vi "Calculate Repeatability.vi"(8 "error in (no error)":errorcluster, 9 "SensorID":i32, 10 "FS Sensors":T1[](array[typedef]), 11 "Calibration Points":T3[](array[typedef])) -> (0 "error out":errorcluster, 2 "Max Repeatability":dbl, 3 "Repeatability Results":T2[](array[typedef]))   [LabVIEW 2026, in "Analysis.lvlib"]
uses:
  Analysis.lvlib
  controls/Messaging Payloads/Calibration Point Table Insert.ctl
  Repeatability Result.ctl
  Full Scale Sensor Cluster.ctl
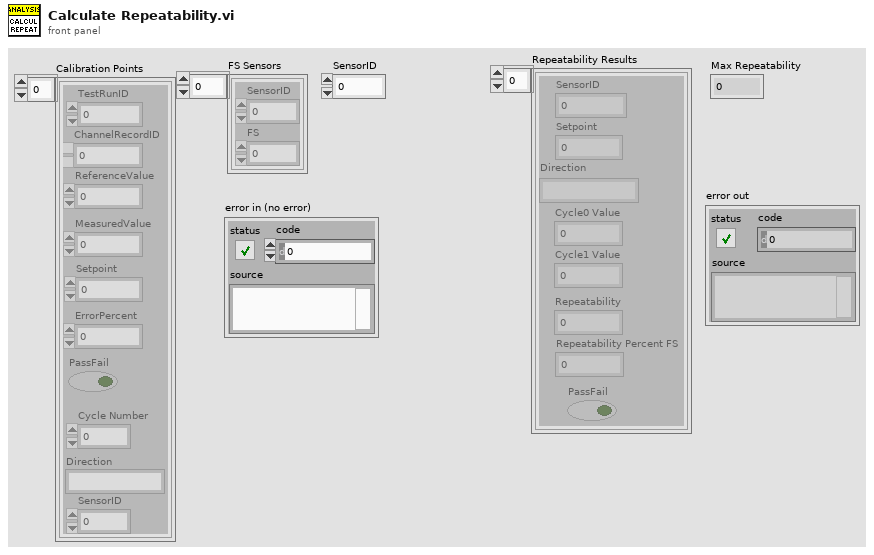
[diagram p1: front panel]
types:
  T1 = typedef "Analysis.lvlib/Full Scale Sensor Cluster.ctl" = cluster{"SensorID":i32, "FS":dbl}
  T2 = typedef "Analysis.lvlib/Repeatability Result.ctl" = cluster{"Setpoint":dbl, "Cycle0 Value":dbl, "SensorID":i32, "Cycle1 Value":dbl, "Repeatability":dbl, "Direction":string, "Repeatability Percent FS":dbl, "PassFail":bool}
  T3 = typedef "Calibration Point Table Insert.ctl" = cluster{"TestRunID":i32, "ChannelRecordID":i32, "Setpoint":dbl, "MeasuredValue":dbl, "ErrorPercent":dbl, "PassFail":bool, "ReferenceValue":dbl, "Cycle Number":i32, "Direction":string, "SensorID":i32}
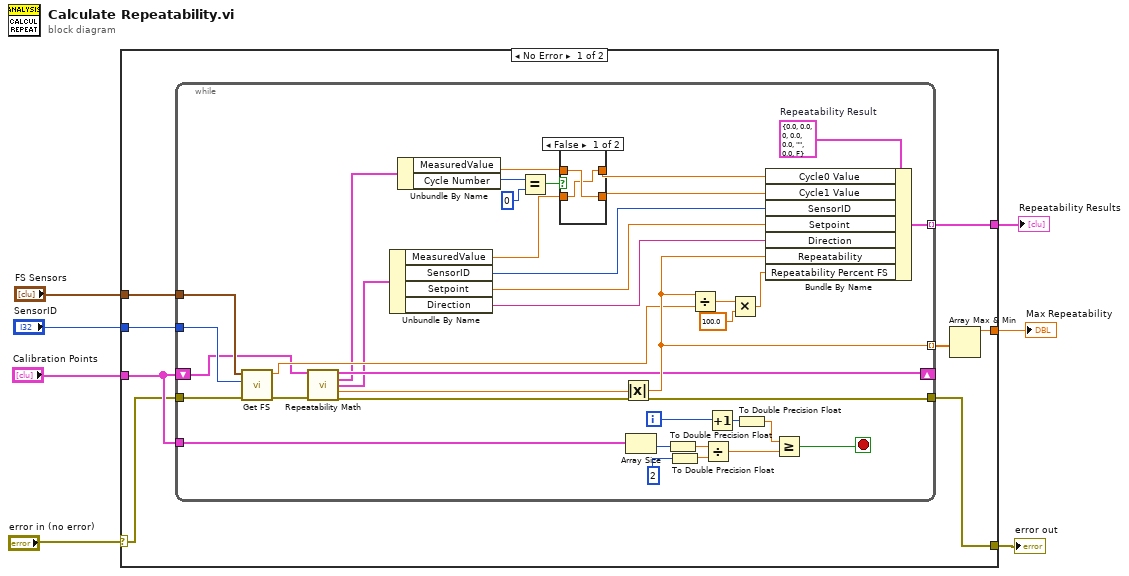
[diagram p0: block diagram]
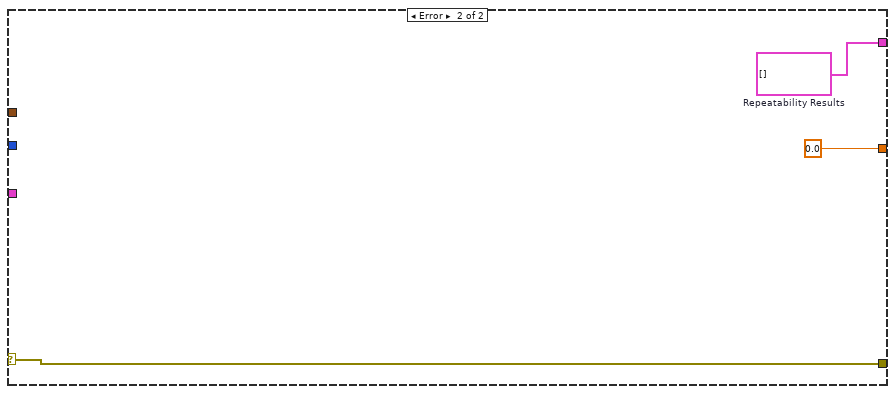
[diagram p3: hidden frame]
diagram:
  n1 = case shown="No Error" "error in (no error)" {
    selector: "error in (no error)" -> [w9 w59]
    tunnel: "Calibration Points" -> [w15 _]
    tunnel: [w8 w59] -> w5
    tunnel: [w14 w58] -> w4
    tunnel: [w12 0.0] -> w3
    tunnel: "FS Sensors" -> [w11 _]
    tunnel: "SensorID" -> [w10 _]
    frame No Error {
      n2 = while {
        shift-right: [w25] -> _
        shift-left: w15 -> [w21]
        tunnel: w15 -> [w43]
        tunnel: [w33] -> w14 mode=indexing
        tunnel: [w27] -> w13 mode=indexing
        tunnel: w11 -> [w32]
        tunnel: w10 -> [w31]
        tunnel: w9 -> [w20]
        tunnel: [w19] -> w8
        i -> [w45]
        stop <- w44 stop-if-true
        w18 = T2 {"Setpoint"=0.0, "Cycle0 Value"=0.0, "SensorID"=0, "Cycle1 Value"=0.0, "Repeatability"=0.0, "Direction"="", "Repeatability Percent FS"=0.0, "PassFail"=FALSE}  # Repeatability Result
        n3 = call "Get FS.vi"("error in (no error)"=w20, "SensorID"=w31, "FS Sensors"=w32) -> ("error out"=w22:errorcluster, "FS"=w26:dbl)  [unwired: 7 in]
        n4 = call "Repeatability Math.vi"("Calibration Points in"=w21, "error in (no error)"=w22) -> ("Calibration Points out"=w25:T3[], "Current Calibration Point"=w24:T3, "Next Calibration Point"=w23:T3, "Numeric"=w42:dbl, "error out"=w19:errorcluster)  [unwired: 9 in]
        n5 = Unbundle By Name(w23) -> ("MeasuredValue"=w34:dbl, "SensorID"=w41:i32, "Setpoint"=w39:dbl, "Direction"=w40:string)
        n6 = Unbundle By Name(w24) -> ("MeasuredValue"=w35:dbl, "Cycle Number"=w38:i32)
        n7 = Equal?(x=w38, y=0) -> (x = y?=w36:bool)
        n8 = case shown="False" w36 {
          tunnel: w35 -> [w54 w56]
          tunnel: [w53 w56] -> w17
          tunnel: w34 -> [w53 w55]
          tunnel: [w54 w55] -> w16
          frame False {
          }
          frame True {
          }
        }
        n9 = Absolute Value(x=w42) -> (abs(x)=w27:dbl)
        n10 = Array Size(array=w43) -> (size(s)=w50:i32)
        n11 = To Double Precision Float(number=w50) -> (double precision float=w49:dbl)
        n12 = To Double Precision Float(number=2 ("index")) -> (double precision float=w47:dbl)
        n13 = Divide(x=w27, y=w26) -> (x/y=w30:dbl)
        n14 = Divide(x=w49, y=w47) -> (x/y=w52:dbl)
        n15 = Increment(x=w45) -> (x+1=w46:i32)
        n16 = Multiply(x=w30, y=100.0) -> (x*y=w28:dbl)
        n17 = To Double Precision Float(number=w46) -> (double precision float=w51:dbl)
        n18 = Bundle By Name(cluster=w18, "Cycle0 Value"=w17, "Cycle1 Value"=w16, "SensorID"=w41, "Setpoint"=w39, "Direction"=w40, "Repeatability"=w27, "Repeatability Percent FS"=w28) -> (w33:T2)
        n19 = Greater Or Equal?(x=w51, y=w52) -> (x >= y?=w44:bool)
      }
      n20 = Array Max & Min(array=w13) -> (max value=w12:dbl)  [unwired: 3 out]
    }
    frame Error {
      w58 = T2[] []  # Repeatability Results
    }
  }
  "error out" <- w5
  "Repeatability Results" <- w4
  "Max Repeatability" <- w3
